vi "Main.vi"() -> ()   [LabVIEW 2015]
uses:
  TypeDefs/Queue Data.ctl
  SubVIs/App Data.vi
  SubVIs/App Strings.vi
  FGV/Timer Actions.ctl
panel:
  in  "Period [s]":dbl
  in  "Device name":tag="myDAQ1"
  out "Time Elapsed":dbl format="%<%M:%S>t"
  out "Status":string
  in  "Time [ms]":dbl
  in  "Frequency":dbl
  in  "Stop Button":bool
  in  "Acquire Button":bool
  out "Waveform Graph":dbl[](graph)
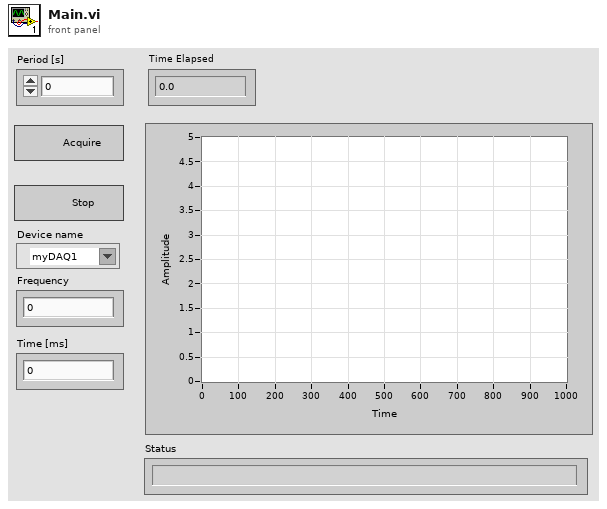
[diagram p1: front panel]
types:
  T1 = typedef "Queue Data.ctl" = cluster{"Action":string}
  T2 = typedef "Timer Actions.ctl" = enum16{"Reset", "Get"}
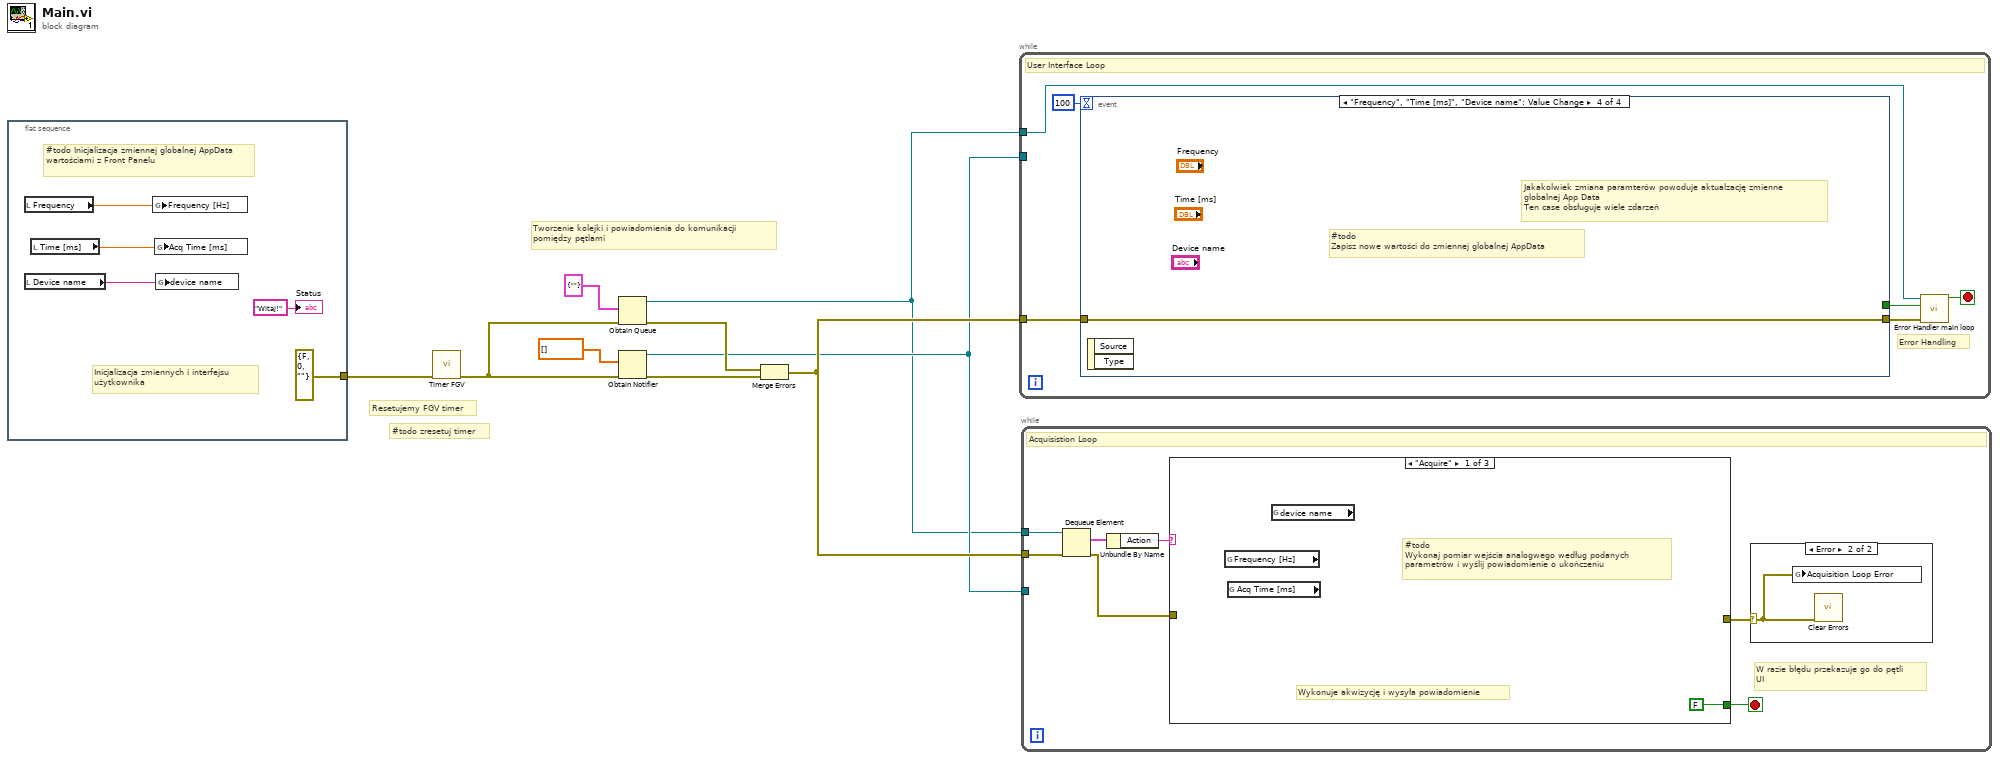
[diagram p0: block diagram]
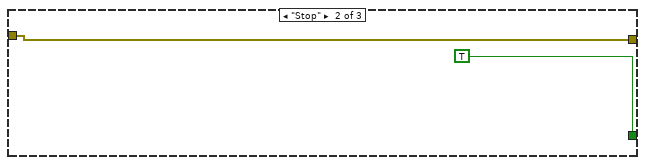
[diagram p3: hidden frame]
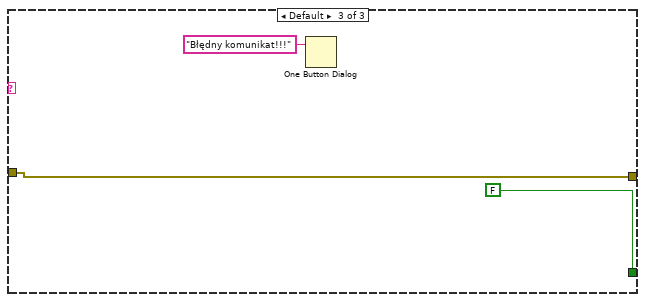
[diagram p4: hidden frame]
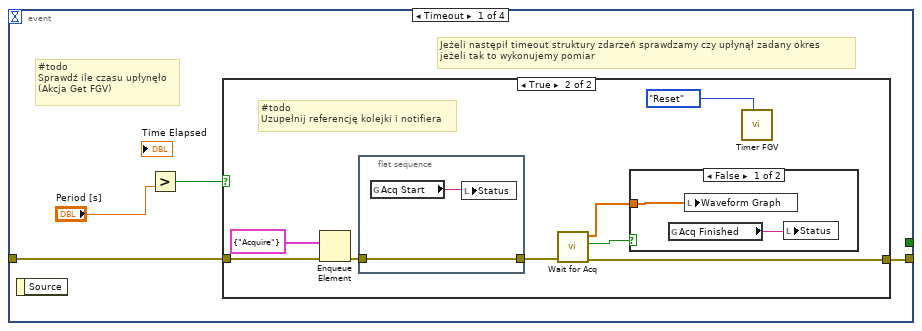
[diagram p5: hidden frame]
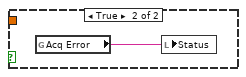
[diagram p7: hidden frame]
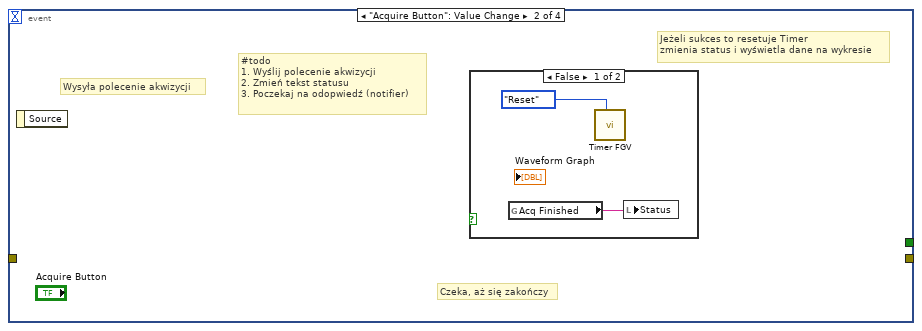
[diagram p8: hidden frame]
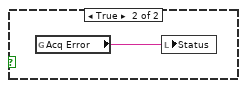
[diagram p9: hidden frame]
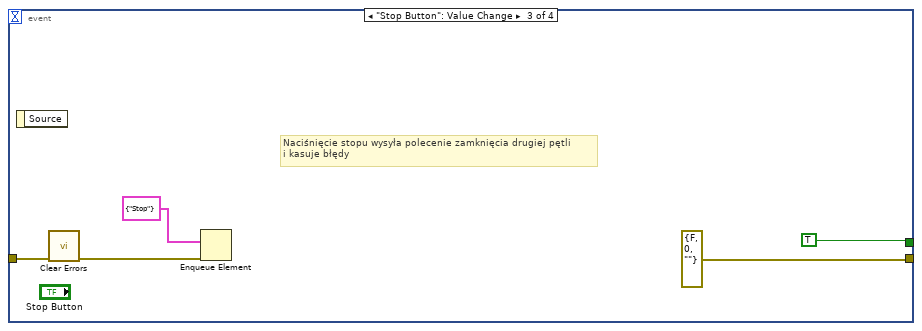
[diagram p10: hidden frame]
diagram:
  # "#todo zresetuj timer"
  # "Resetujemy FGV timer"
  # "Tworzenie kolejki i powiadomienia do komunikacji \npomiędzy pętlami"
  n1 = flat-sequence {
    tunnel: [errorcluster {"status"=FALSE, "code"=0, "source"=""} ("error constant")] -> w2
    frame #0 {
      # "#todo Inicjalizacja zmiennej globalnej AppData wartościami z Front Panelu"
      # "Inicjalizacja zmiennych i interfejsu \nużytkownika"
      n2 = local read "Frequency"() -> (w12:dbl)
      n3 = local read "Device name"() -> (w10:tag)
      n4 = local read "Time [ms]"() -> (w11:dbl)
      n5 = global write "App Data.vi" "Frequency [Hz]"(w12) -> ()
      n6 = global write "App Data.vi" "Acq Time [ms]"(w11) -> ()
      n7 = global write "App Data.vi" "device name"(w10) -> ()
      "Status" <- "Witaj!" ("Status")
    }
  }
  n8 = call "Timer FGV.vi"("error in (no error)"=w2) -> ("error out"=w1:errorcluster)  [unwired: 9 in, 1 out]
  n9 = Obtain Queue(element data type=T1 {"Action"=""}, error in (no error)=w1) -> (queue out=w3:refnum<queue>, error out=w8:errorcluster)  [unwired: 3 in, 1 out]
  n10 = Obtain Notifier(notification data type=dbl[] [], error in (no error)=w1) -> (notifier out=w4:refnum<notifier>, error out=w6:errorcluster)  [unwired: 2 in, 1 out]
  n11 = Merge Errors(w8, w6) -> (w5:errorcluster)
  n12 = while {
    tunnel: w5 -> [w19]
    tunnel: w3 -> [w15]
    tunnel: w4 -> [_]
    stop <- w16 stop-if-true
    # "Error Handling"
    # "User Interface Loop"
    n13 = event shown="[3] \"Frequency\", \"Time [ms]\", \"Device name\": Value Change" {
      selector: _ -> [_ _ _ _]
      dyn-events: _ -> [_ _ _ _]
      timeout: 100 -> [_ _ _ _]
      tunnel: w19 -> [w22 _ w43 w47]
      tunnel: [w21 _ errorcluster {"status"=FALSE, "code"=0, "source"=""} ("error constant") w47] -> w17
      tunnel: [_ _ TRUE _] -> w18
      event Timeout {
        # "#todo\nSprawdź ile czasu upłynęło\n(Akcja Get FGV)"
        # "Jeżeli następił timeout struktury zdarzeń sprawdzamy czy upłynął zadany okres \njeżeli tak to wykonujemy pomiar"
        n14 = event-data() -> ()  [unwired: 1 in, 1 out]
        n15 = Greater?(y="Period [s]") -> (0:w23:bool)  [unwired: 1 in]
        n16 = case shown="True" w23 {
          tunnel: w22 -> [w25 w33]
          tunnel: [w25 w26] -> w21
          frame False {
          }
          frame True {
            # "#todo\nUzupełnij referencję kolejki i notifiera"
            n17 = Enqueue Element(element=T1 {"Action"="Acquire"}, error in (no error)=w33) -> (error out=w31:errorcluster)  [unwired: 2 in, 2 out]
            n18 = flat-sequence {
              tunnel: w31 -> [w37]
              tunnel: [w37] -> w30
              frame #0 {
                n19 = global read "App Strings.vi" "Acq Start"() -> (w38:string)
                n20 = local write "Status"(w38) -> ()
              }
            }
            n21 = call "Wait for Acq.vi"("error in (no error)"=w30) -> ("error out"=w26:errorcluster, "timed out?"=w27:bool, "Array"=w29:dbl[])  [unwired: 8 in]
            n22 = case shown="False" w27 {
              tunnel: w29 -> [w34 _]
              frame False {
                n23 = global read "App Strings.vi" "Acq Finished"() -> (w35:string)
                n24 = local write "Waveform Graph"(w34) -> ()
                n25 = local write "Status"(w35) -> ()
              }
              frame True {
                n26 = global read "App Strings.vi" "Acq Error"() -> (w36:string)
                n27 = local write "Status"(w36) -> ()
              }
            }
            n28 = call "Timer FGV.vi"("Action"=Timer_Actions."Reset") -> ()  [unwired: 9 in, 2 out]
          }
        }
      }
      event "Acquire Button": Value Change {
        # "#todo\n1. Wyślij polecenie akwizycji\n2. Zmień tekst statusu\n3. Poczekaj na odopwiedź (notifier)"
        # "Jeżeli sukces to resetuje Timer\nzmienia status i wyświetla dane na wykresie"
        # "Czeka, aż się zakończy"
        # "Wysyła polecenie akwizycji"
        n29 = event-data() -> ()  [unwired: 1 in, 1 out]
        n30 = case shown="False" {
          selector: _ -> [_ _]
          frame False {
            n31 = global read "App Strings.vi" "Acq Finished"() -> (w40:string)
            n32 = call "Timer FGV.vi"("Action"=Timer_Actions."Reset") -> ()  [unwired: 9 in, 2 out]
            n33 = local write "Status"(w40) -> ()
          }
          frame True {
            n34 = global read "App Strings.vi" "Acq Error"() -> (w41:string)
            n35 = local write "Status"(w41) -> ()
          }
        }
      }
      event "Stop Button": Value Change {
        # "Naciśnięcie stopu wysyła polecenie zamknięcia drugiej pętli\ni kasuje błędy"
        n36 = event-data() -> ()  [unwired: 1 in, 1 out]
        n37 = call <vilib>:"Clear Errors.vi"("error in (no error)"=w43) -> ("error out"=w42:errorcluster)  [unwired: 5 in, 1 out]
        n38 = Enqueue Element(element=T1 {"Action"="Stop"}, error in (no error)=w42) -> ()  [unwired: 2 in, 3 out]
      }
      event "Frequency", "Time [ms]", "Device name": Value Change {
        # "#todo \nZapisz nowe wartości do zmiennej globalnej AppData"
        # "Jakakolwiek zmiana paramterów powoduje aktualzację zmienne \nglobalnej App Data\nTen case obsługuje wiele zdarzeń"
        n39 = event-data() -> ()  [unwired: 1 in, 2 out]
      }
    }
    n40 = call "Error Handler main loop.vi"("error in (no error)"=w17, "Exit?"=w18, "Queue in"=w15) -> ("Exit?"=w16:bool)  [unwired: 8 in]
  }
  n41 = while {
    tunnel: w5 -> [w52]
    tunnel: w3 -> [w51]
    tunnel: w4 -> [_]
    stop <- w49 stop-if-true
    # "W razie błędu przekazuje go do pętli\nUI"
    # "Acquisistion Loop"
    n42 = Dequeue Element(queue=w51, error in (no error)=w52) -> (element=w54:T1, error out=w50:errorcluster)  [unwired: 1 in, 2 out]
    n43 = Unbundle By Name(w54) -> ("Action"=w53:string)
    n44 = case shown="\"Acquire\"" w53 {
      tunnel: w50 -> [_ w57 w60]
      tunnel: [FALSE TRUE FALSE] -> w49
      tunnel: [_ w57 w60] -> w48
      frame "Acquire" {
        # "#todo\nWykonaj pomiar wejścia analogwego według podanych \nparametrów i wyślij powiadomienie o ukończeniu"
        # "Wykonuje akwizycję i wysyła powiadomienie"
        n45 = global read "App Data.vi" "Frequency [Hz]"() -> ()  [unwired: 1 out]
        n46 = global read "App Data.vi" "Acq Time [ms]"() -> ()  [unwired: 1 out]
        n47 = global read "App Data.vi" "device name"() -> ()  [unwired: 1 out]
      }
      frame "Stop" {
      }
      frame Default {
        n48 = One Button Dialog(message="Błędny komunikat!!!") -> ()  [unwired: 1 in, 1 out]
      }
    }
    n49 = case shown="Error" w48 {
      selector: w48 -> [_ w55]
      frame No Error {
      }
      frame Error {
        n50 = global write "App Data.vi" "Acquisition Loop Error"(w55) -> ()
        n51 = call <vilib>:"Clear Errors.vi"("error in (no error)"=w55) -> ()  [unwired: 5 in, 2 out]
      }
    }
  }
